vi "lasers pew pew (2).vi"() -> ()   [LabVIEW 2016]
uses:
  <vilib>/DAQmx/read.llb/DAQmx Read (Analog DBL 1Chan 1Samp).vi
  <vilib>/DAQmx/miscellaneous.llb/DAQmx Fill In Error Info.vi
panel:
  in  "Output kW from Request":dbl
  out "Combined Readings":dbl
  in  "stop":bool
  in  "Requested kW":dbl
  out "Difference Btwn Predictions":dbl
  out "Waveform Chart":dbl[](graph)
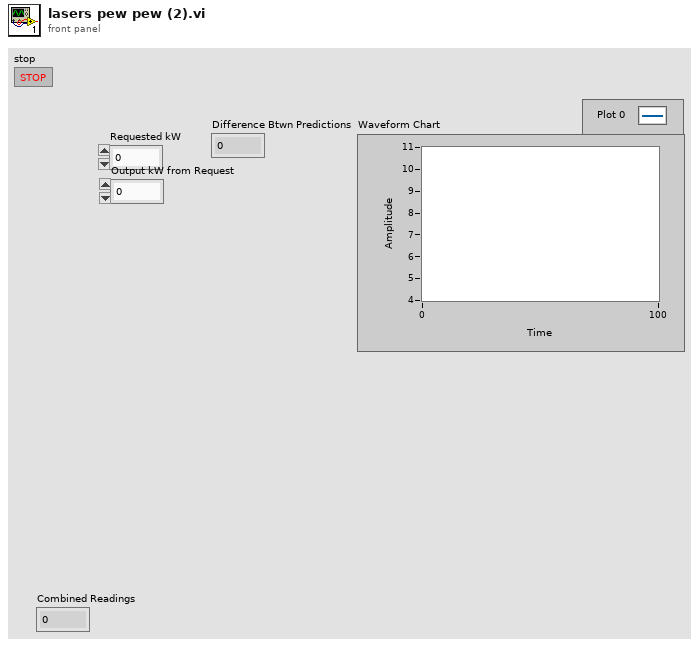
[diagram p1: front panel]
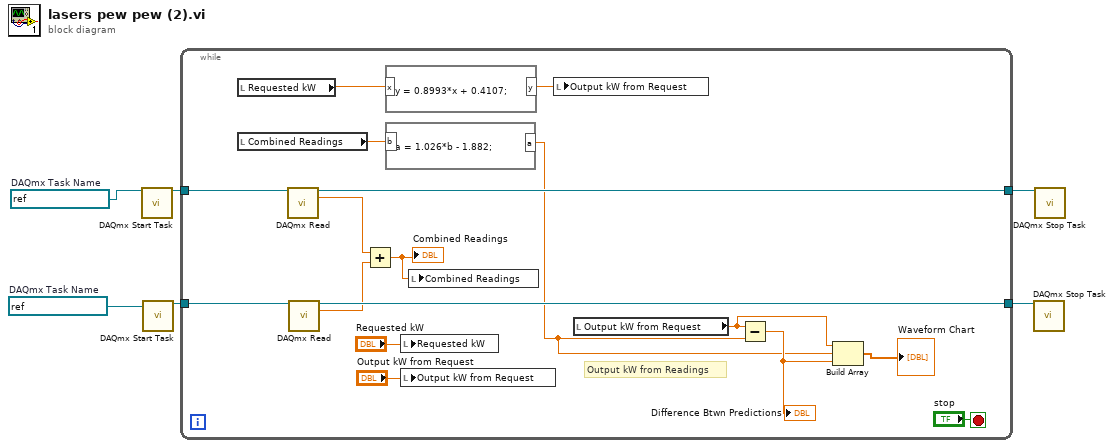
[diagram p0: block diagram]
diagram:
  w5 = refnum<k21> "Laser3_Power"  # DAQmx Task Name
  w6 = refnum<k21> "Laser2_Power"  # DAQmx Task Name
  n1 = call <vilib>:"DAQmx Start Task.vi"("task/channels in"=w6) -> ("task out"=w4:refnum<k21>)  [unwired: 13 in, 1 out]
  n2 = call <vilib>:"DAQmx Start Task.vi"("task/channels in"=w5) -> ("task out"=w3:refnum<k21>)  [unwired: 13 in, 1 out]
  n3 = while {
    tunnel: w4 -> [w19]
    tunnel: w3 -> [w18]
    tunnel: [w17] -> w2
    tunnel: [w16] -> w1
    stop <- "stop" stop-if-true
    # "Output kW from Readings"
    n4 = local read "Requested kW"() -> (w13:dbl)
    n5 = local read "Combined Readings"() -> (w12:dbl)
    n6 = call-poly <vilib>:"DAQmx Read.vi"("task/channels in"=w19) -> ("task out"=w16:refnum<k21>, "data"=w14:dbl)  [unwired: 12 in, 1 out]
    n7 = call-poly <vilib>:"DAQmx Read.vi"("task/channels in"=w18) -> ("task out"=w17:refnum<k21>, "data"=w15:dbl)  [unwired: 12 in, 1 out]
    n8 = Add(x=w14, y=w15) -> (x+y=w20:dbl)
    "Combined Readings" <- w20
    n9 = formula code="y = 0.8993*x + 0.4107;"("x"=w13) -> ("y"=w10:dbl)
    n10 = formula code="a = 1.026*b - 1.882;"("b"=w12) -> ("a"=w7:dbl)
    n11 = local write "Requested kW"("Requested kW") -> ()
    n12 = local write "Output kW from Request"("Output kW from Request") -> ()
    n13 = local write "Combined Readings"(w20) -> ()
    n14 = local write "Output kW from Request"(w10) -> ()
    n15 = local read "Output kW from Request"() -> (w9:dbl)
    n16 = Subtract(x=w9, y=w7) -> (x-y=w8:dbl)
    "Difference Btwn Predictions" <- w8
    n17 = Build Array(w9, w7, w8) -> (→"Waveform Chart":dbl[])
  }
  n18 = call <vilib>:"DAQmx Stop Task.vi"("task/channels in"=w2) -> ()  [unwired: 13 in, 2 out]
  n19 = call <vilib>:"DAQmx Stop Task.vi"("task/channels in"=w1) -> ()  [unwired: 13 in, 2 out]
